vi "getRequirements.vi"(8 "error in (no error)":errorcluster, 10 "Active Item:Tag":string, 11 "Tree Control":refnum<vi>) -> (0 "error out":errorcluster, 2 "Requirements":string[](array[string]), 3 "Tree Control out":refnum<vi>)   [LabVIEW 2010]
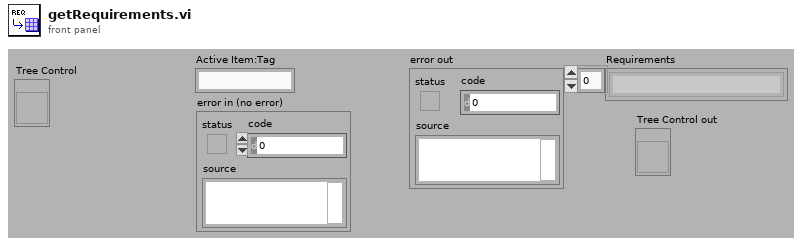
[diagram p1: front panel]
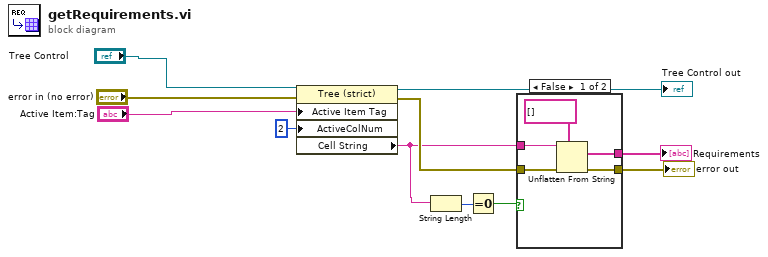
[diagram p0: block diagram]
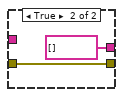
[diagram p2: hidden frame]
diagram:
  n1 = property class="Tree (strict)"(reference="Tree Control", error in="error in (no error)", "Active Item Tag"="Active Item:Tag", "ActiveColNum"=2 ("Active Cell:Active Column Number")) -> (reference out=→"Tree Control out":refnum<vi>, error out=w8:errorcluster, "Cell String"=w3:string)
  n2 = String Length(string=w3) -> (length=w2:i32)
  n3 = Equal To 0?(x=w2) -> (x = 0?=w1:bool)
  n4 = case shown="False" w1 {
    tunnel: w8 -> [w15 w18]
    tunnel: [w14 w18] -> w7
    tunnel: [w13 string[] []] -> w6
    tunnel: w3 -> [w12 _]
    frame False {
      n5 = Unflatten From String(type=string[] [], binary string=w12, error in (no error)=w15) -> (value=w13:string[], error out=w14:errorcluster)  [unwired: 2 in, 1 out]
    }
    frame True {
    }
  }
  "error out" <- w7
  "Requirements" <- w6
